vi "Kinesis - KNA - Latch Trak.vi"() -> ()   [LabVIEW 2015]
doc: "Shows how to set the NanoTrak Latch and Trak mode."
uses:
  C:/Users/fmovagharnemati/OneDrive - THORLABS Inc/Desktop/Kinesis_with_LabVIEW_Examples_LV12 - v3/Thorlabs.MotionControl.Controls.dll
  Thorlabs.MotionControl.Controls.dll
  C:/Users/fmovagharnemati/OneDrive - THORLABS Inc/Desktop/Kinesis_with_LabVIEW_Examples_LV12 - v3/Thorlabs.MotionControl.KCube.NanoTrakCLI.dll
  Thorlabs.MotionControl.KCube.NanoTrakCLI.dll
panel:
  in  "SerialNumber":string
  in  "?":bool
  in  "?":bool
  in  "?":bool
  in  "KCubeNanoTrakControl":refnum<k24>(container)
  # "Notes:"
  # "- Ensure that the appropriate .DLLs are copied into your Project Folder. Check that the correct bit type are used depending on your version of LabVIEW\ni.e. 32-bit or 64-bit.\n\n\n\n\n\n\n\n\n\n\n\n\n\n\n- Open the example VI through the LabVIEW Project Explorer to correctly load the User Interface from Thorlabs.MotionControl.Controls.dll."
  # "Thorlabs Hardware: KNA - K-Cube Nanotrak Controller\nhttps://www.thorlabs.com/newgrouppage9.cfm?objectgroup_id=2877"
  # "Description: This VI will enable you to run the Kinesis Device panel for KNA-nnn devices. \nYou will also be able to set the Operating Mode to Track or Latch.\n\nTrack - When tracking, the NanoTrak detects any drop in signal strength resulting from misalignment of the input and output devices, and makes positional adjustments to maintain the maximum signal strength.\n\nLatch - Scanning is disabled and the piezo drives are held at their present position.\n\n1. Connect your KNA-nnn device to your PC via USB & power your device.\n2. Enter the serial number of the controller into the SerialNumber box below.\n3. Run the VI"
  # "Example Image of .NET Controller - VI opened via Project Explorer/ not opened via Project Explorer"
  # "VI Not Opened via Project Explorer"
  # "VI Opened via Project Explorer"
  # "- To explore the range of methods available, please visit the .NET API, included with your Kinesis software.\n\n- For tips on building your own VIs with Thorlabs Motion Control Hardware, please see our LabVIEW Guide here.\nhttps://www.thorlabs.com/newgrouppage9.cfm?objectgroup_id=10285"
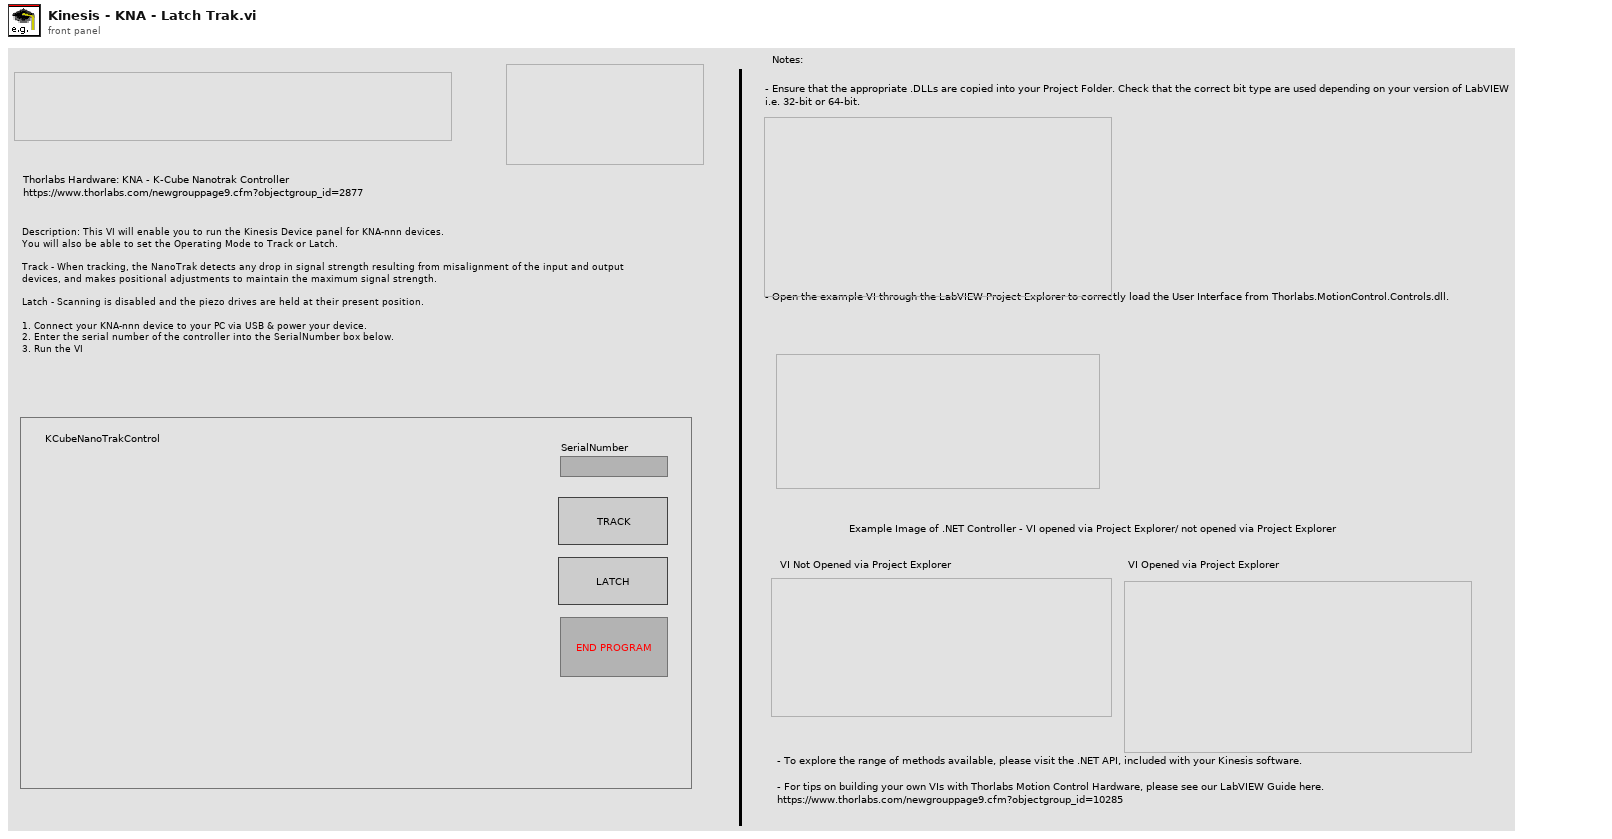
[diagram p1: front panel]
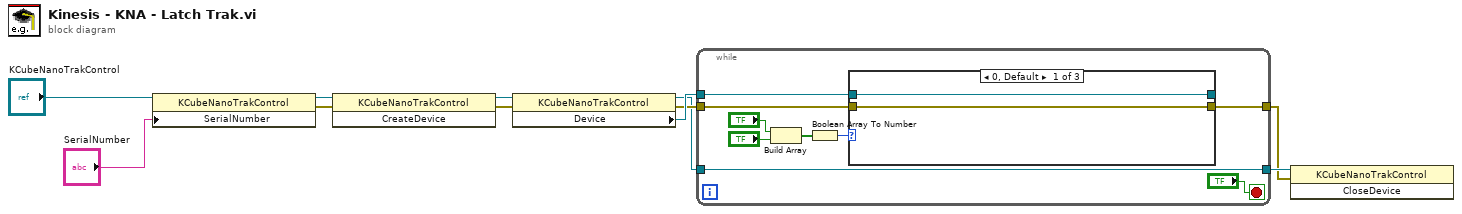
[diagram p0: block diagram]
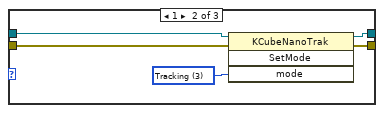
[diagram p2: hidden frame]
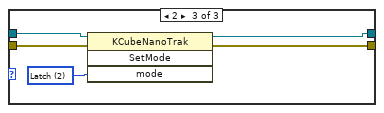
[diagram p3: hidden frame]
diagram:
  n1 = property class="KCubeNanoTrakControl"(reference="KCubeNanoTrakControl", "SerialNumber"="SerialNumber") -> (reference out=w9:refnum<k24>, error out=w8:errorcluster)  [unwired: 1 in]
  n2 = invoke class="KCubeNanoTrakControl" method="CreateDevice"(reference=w9, error in=w8) -> (reference out=w11:refnum<k24>, error out=w10:errorcluster)  [unwired: 1 in, 1 out]
  n3 = property class="KCubeNanoTrakControl"(reference=w11, error in=w10) -> (reference out=w2:refnum<k24>, error out=w4:errorcluster, "Device"=w6:refnum<k24>)
  n4 = while {
    tunnel: w6 -> [w15]
    tunnel: w4 -> [w14]
    tunnel: [w13] -> w3
    tunnel: w2 -> [w13]
    tunnel: [w12] -> w1
    stop <- "?" stop-if-true
    n5 = Build Array("?", "?") -> (w18:bool[])
    n6 = Boolean Array To Number(Boolean array=w18) -> (number=w17:u32)
    n7 = case shown="0, Default" w17 {
      tunnel: [w22 w26 w30] -> _
      tunnel: w15 -> [w22 w27 w31]
      tunnel: w14 -> [w21 w24 w29]
      tunnel: [w21 w23 w28] -> w12
      frame 0, Default {
      }
      frame 1 {
        w25 = 3 items=["Undefined", "Piezo", "Latch", "Tracking", "HorizontalTracking", "VerticalTracking"] ("mode")
        n8 = invoke class="KCubeNanoTrak" method="SetMode"(reference=w27, error in=w24, "mode"=w25) -> (reference out=w26:refnum<k24>, error out=w23:errorcluster)  [unwired: 1 in, 2 out]
      }
      frame 2 {
        w32 = 2 items=["Undefined", "Piezo", "Latch", "Tracking", "HorizontalTracking", "VerticalTracking"] ("mode")
        n9 = invoke class="KCubeNanoTrak" method="SetMode"(reference=w31, error in=w29, "mode"=w32) -> (reference out=w30:refnum<k24>, error out=w28:errorcluster)  [unwired: 1 in, 2 out]
      }
    }
  }
  n10 = invoke class="KCubeNanoTrakControl" method="CloseDevice"(reference=w3, error in=w1) -> ()  [unwired: 1 in, 3 out]
